vi "Event_ball_region.vi"(8 "error in (no error)":errorcluster, 10 "Game in":refnum<class "Game.lvclass">, 11 "Events in":refnum<class "Events.lvclass">) -> (0 "error out":errorcluster, 3 "Events out":refnum<class "Events.lvclass">)   [LabVIEW 2023, in "Events.lvclass"]
uses:
  Events.lvclass
  Game_class/Game.lvclass
  Game_class/Game.lvclass/Game.ctl
  Object_class/Object.lvclass/Object.ctl
  Game_class/Read BallRef.vi
  Object_class/Read position(x,y).vi
  Ball_class/Ball.lvclass
  C:/Users/ebert/Desktop/roboime/SSL_AI/Object_class/Object.lvclass
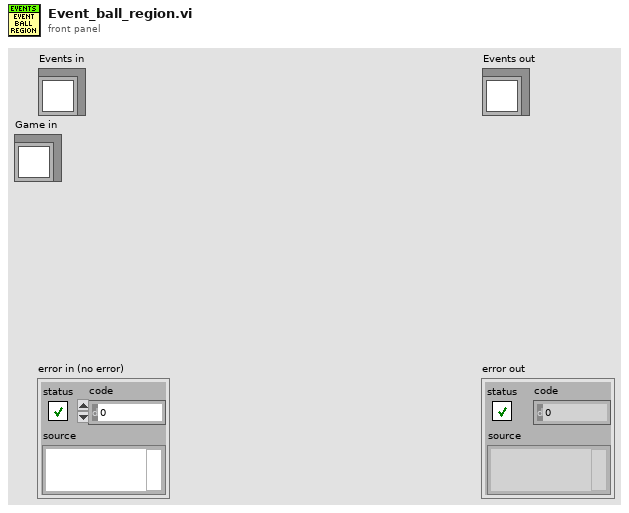
[diagram p1: front panel]
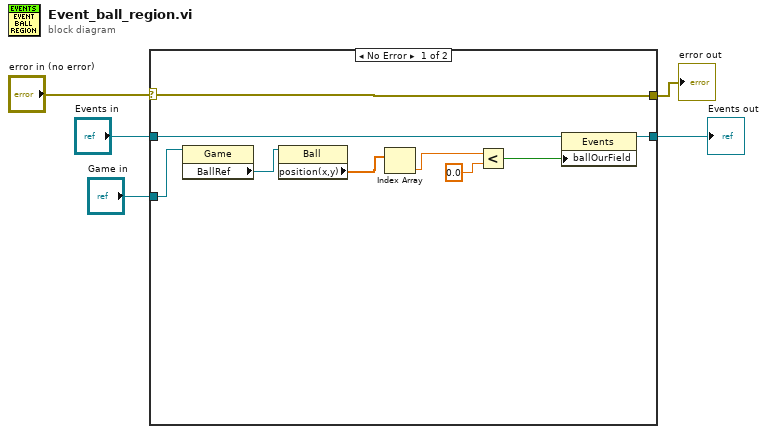
[diagram p0: block diagram]
diagram:
  n1 = case shown="No Error" "error in (no error)" {
    selector: "error in (no error)" -> [w14 w16]
    tunnel: [w14 w16] -> w4
    tunnel: [w12 w15] -> w2
    tunnel: "Events in" -> [w13 w15]
    tunnel: "Game in" -> [w9 _]
    frame No Error {
      n2 = property class="Game"(reference=w9) -> ("BallRef"=w8:refnum<class "Ball.lvclass">)  [unwired: 1 in, 2 out]
      n3 = property class="Ball"(reference=w8) -> ("position(x,y)"=w6:dbl[])  [unwired: 1 in, 2 out]
      n4 = Index Array(array=w6) -> (element=w7:dbl)  [unwired: 1 in]
      n5 = Less?(x=w7, y=0.0) -> (x < y?=w10:bool)
      n6 = property class="Events"(reference=w13, "ballOurField"=w10) -> (reference out=w12:refnum<class "Events.lvclass">)  [unwired: 1 in, 1 out]
    }
    frame Error {
    }
  }
  "error out" <- w4
  "Events out" <- w2
